vi "数字输出_软件按需单点(多线).vi"() -> ()   [LabVIEW 2013]
doc: "This example demonstrates how to output voltage from multi digital lines(channels)."
uses:
  <userlib>/ArtDAQ/_SubVI/ArtDAQ_CreateDOChan.vi
  <userlib>/ArtDAQ/_SubVI/ArtDAQ_Write Digital U32 1Chan 1Samp.vi
panel:
  in  "Data":bool[](array[boolean])=[TRUE, TRUE, FALSE]
  out "错误输出":errorcluster
  in  "线通道":string="Dev1/port0/line0:2"
  in  "Stop":bool
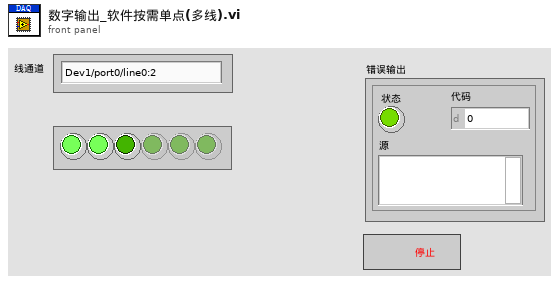
[diagram p1: front panel]
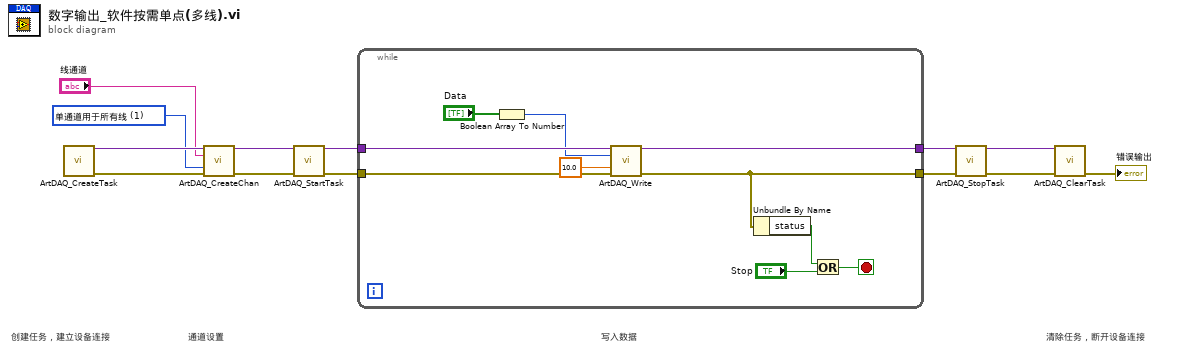
[diagram p0: block diagram]
diagram:
  w3 = 1 items=["单通道用于单条线", "单通道用于所有线"] ("Line Grouping")
  # "清除任务，断开设备连接"
  # "写入数据"
  # "通道设置"
  # "创建任务，建立设备连接"
  n1 = call <userlib>:"ArtDAQ_CreateTask.vi"() -> ("任务句柄"=w13:variant, "错误输出"=w12:errorcluster)  [unwired: 14 in]
  n2 = call-poly <userlib>:"ArtDAQ_CreateChan.vi"("任务句柄"=w13, "线"="线通道", "线分组"=w3, "错误输入"=w12) -> ("任务句柄"=w11:variant, "错误输出"=w10:errorcluster)  [unwired: 10 in]
  n3 = call <userlib>:"ArtDAQ_StartTask.vi"("任务句柄"=w11, "错误输入"=w10) -> ("任务句柄"=w9:variant, "错误输出"=w8:errorcluster)  [unwired: 12 in]
  n4 = while {
    tunnel: w9 -> [w23]
    tunnel: w8 -> [w22]
    tunnel: [w21] -> w7
    tunnel: [w20] -> w6
    stop <- w18 stop-if-true
    n5 = Boolean Array To Number(Boolean array="Data") -> (number=w14:u32)
    n6 = call-poly <userlib>:"ArtDAQ_Write.vi"("任务句柄"=w23, "数据"=w14, "超时s"=10.0 ("Timeout"), "错误输入"=w22) -> ("任务句柄"=w21:variant, "错误输出"=w20:errorcluster)  [unwired: 10 in]
    n7 = Unbundle By Name(w20) -> ("status"=w19:bool)
    n8 = Or(x=w19, y="Stop") -> (x .or. y?=w18:bool)
  }
  n9 = call <userlib>:"ArtDAQ_StopTask.vi"("任务句柄"=w7, "错误输入"=w6) -> ("任务句柄"=w5:variant, "错误输出"=w4:errorcluster)  [unwired: 12 in]
  n10 = call <userlib>:"ArtDAQ_ClearTask.vi"("任务句柄"=w5, "错误输入"=w4) -> ("错误输出"=→"错误输出":errorcluster)  [unwired: 13 in]
